vi "sv_Harmonic Magnitude and Phase Plot (XY).vi"(8 "speed profile":T1 {"speed [RPM]" format="%.2f"; "time [s]" format="%.2f"}, 10 "phase lag  (even angular)":dbl[][][](array[numeric]) format="%.2f", 11 "magnitudes (even angular)":dbl[][][](array[numeric]) format="%.2f") -> (1 "X unit":string, 2 "phase lag":cluster{"X":dbl[], "Y":dbl[]}[][](array[cluster]) {"Y" format="%.2f"; "X" format="%.2f"}, 3 "magnitudes":cluster{"X":dbl[], "Y":dbl[]}[][](array[cluster]) {"Y" format="%.2f"; "X" format="%.2f"})   [LabVIEW 2017, in "SoundVib_ContSweptSine.lvlib"]
uses:
  <vilib>/addons/Sound and Vibration/svt_Continuous Swept Sine/SoundVib_ContSweptSine.lvlib
  <vilib>/addons/Sound and Vibration/Order Analysis/Tach Process/SubVIs/speed profile.ctl
  <vilib>/addons/Sound and Vibration/Order Analysis/Tach Process/SoundVib_TachProcess.lvlib
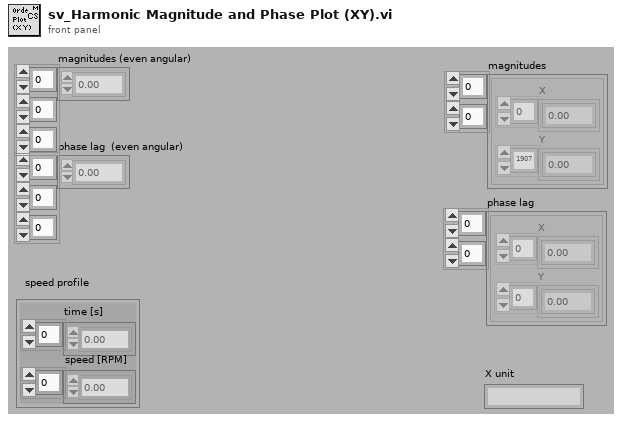
[diagram p1: front panel]
types:
  T1 = typedef "SoundVib_TachProcess.lvlib/speed profile.ctl" = cluster{"time [s]":dbl[], "speed [RPM]":dbl[]}
  T2 = cluster{dbl[], "magnitudes (even angular)":dbl[]}
  T3 = cluster{dbl[], "phase lag  (even angular)":dbl[]}
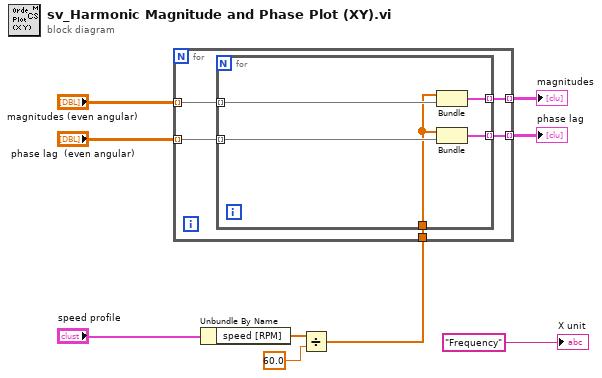
[diagram p0: block diagram]
diagram:
  n1 = Unbundle By Name("speed profile") -> ("speed [RPM]"=w2:dbl[])
  n2 = Divide(x=w2, y=60.0) -> (x/y=w6:dbl[])
  n3 = for {
    tunnel: "magnitudes (even angular)" -> [w14] mode=indexing
    tunnel: "phase lag  (even angular)" -> [w13] mode=indexing
    tunnel: w6 -> [w12]
    tunnel: [w11] -> w4 mode=indexing
    tunnel: [w10] -> w3 mode=indexing
    n4 = for {
      tunnel: w13 -> [w16] mode=indexing
      tunnel: [w18] -> w10 mode=indexing
      tunnel: [w19] -> w11 mode=indexing
      tunnel: w14 -> [w17] mode=indexing
      tunnel: w12 -> [w15]
      n5 = Bundle(w15, "magnitudes (even angular)"=w17) -> (w19:T2)  [unwired: 1 out]
      n6 = Bundle(w15, "phase lag  (even angular)"=w16) -> (w18:T3)  [unwired: 1 out]
    }
  }
  "phase lag" <- w3
  "magnitudes" <- w4
  "X unit" <- "Frequency"
